vi "SCMP CoMP-S Mechanism - Diffuser.vi"(8 "error in (no error)":errorcluster, 9 "Auto Motors":bool, 10 "Old Diffuser":T1=enum."In Beam", 11 "Desired Diffuser":T1=enum."In Beam") -> (0 "error out":errorcluster, 3 "New Diffuser":T1=enum."In Beam")   [LabVIEW 2014]
uses:
  Controls/Diffuser.ctl
panel:
  # "Moving Diffuser\n    wait please"
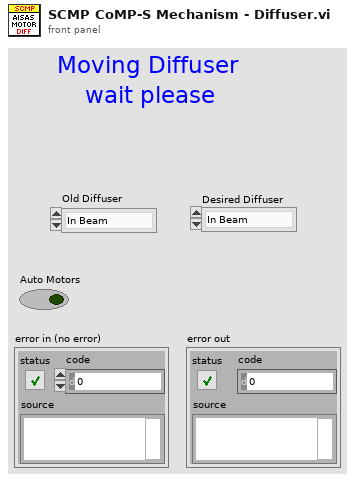
[diagram p1: front panel]
types:
  T1 = typedef "Diffuser.ctl" = enum16{"Out of Beam", "In Beam"}
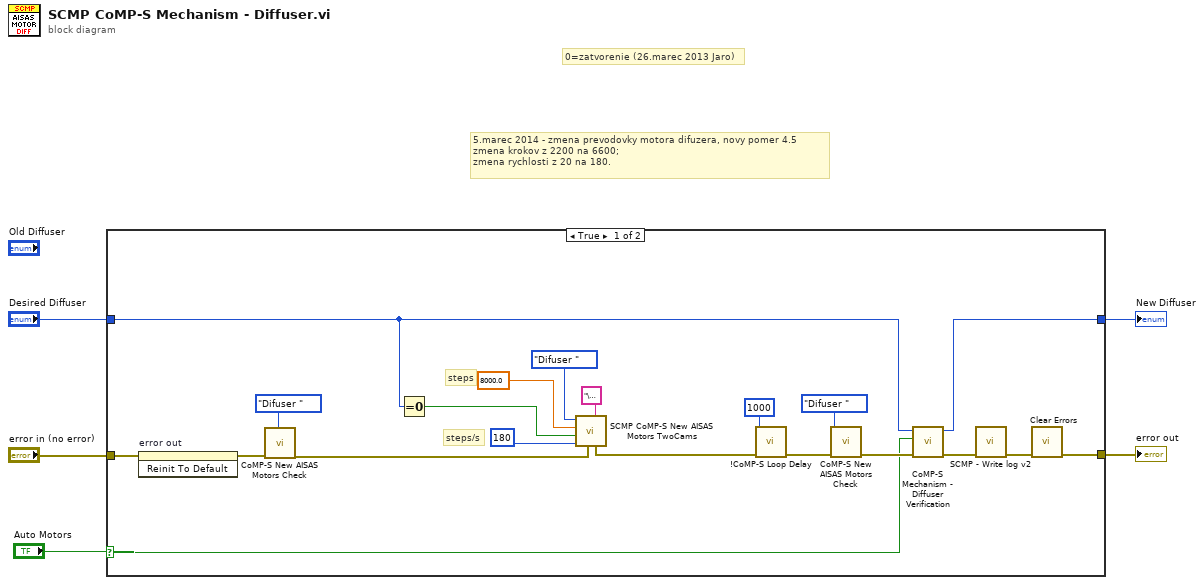
[diagram p0: block diagram]
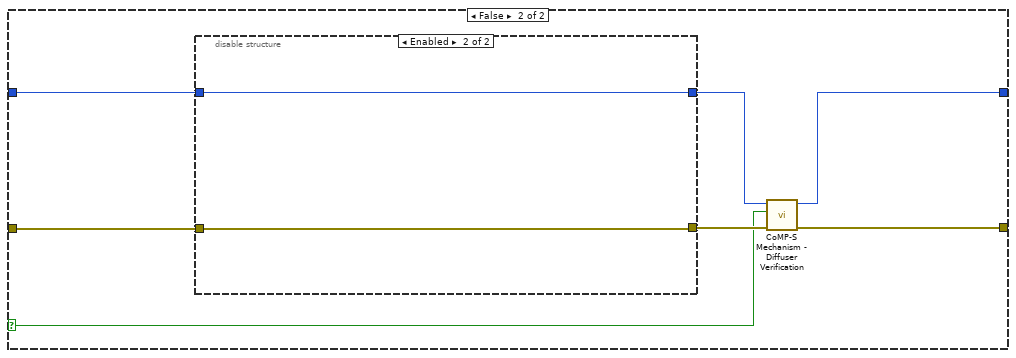
[diagram p2: hidden frame]
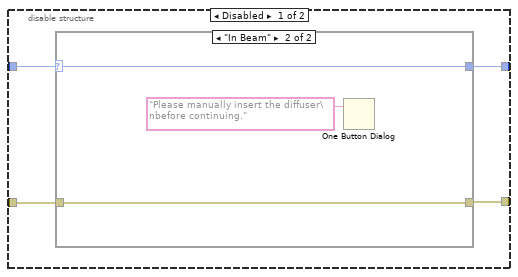
[diagram p3: hidden frame]
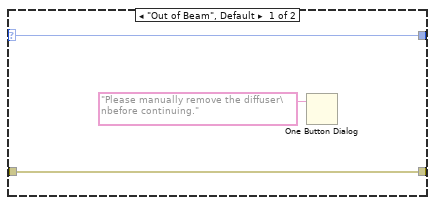
[diagram p4: hidden frame]
diagram:
  # "0=zatvorenie (26.marec 2013 Jaro)"
  # "5.marec 2014 - zmena prevodovky motora difuzera, novy pomer 4.5\nzmena krokov z 2200 na 6600;\nzmena rychlosti z 20 na 180."
  n1 = case shown="True" "Auto Motors" {
    selector: "Auto Motors" -> [w18 w26]
    tunnel: "error in (no error)" -> [w17 w32]
    tunnel: [w13 w29] -> w3
    tunnel: [w15 w27] -> w1
    tunnel: "Desired Diffuser" -> [w7 w31]
    frame True {
      # "steps/s"
      # "steps"
      n2 = invoke on="error out" class="Clust (strict)" method="Reinit To Default"(error in=w17) -> (error out=w16:errorcluster)  [unwired: 2 in, 2 out]
      n3 = call "CoMP-S New AISAS Motors Check.vi"("error in (no error)"=w16, "Motor selection"=enum32{"Rotation", "Difuser ", "Objective Lens"}."Difuser ") -> ("error out"=w20:errorcluster)  [unwired: 9 in]
      n4 = Equal To 0?(x=w7) -> (x = 0?=w6:bool)
      n5 = call "SCMP CoMP-S New AISAS Motors TwoCams.vi"("Motion Code"="\u0002", "error in (no error)"=w20, "steps/sec"=u32 180, "motor rotation"=w6, "Steps"=8000.0, "Motor selection"=enum32{"Rotation", "Difuser ", "Objective Lens"}."Difuser ") -> ("error out"=w21:errorcluster)  [unwired: 2 in, 3 out]
      n6 = call "!CoMP-S Loop Delay.vi"("error in (no error)"=w21, "Delay (2000ms)"=1000) -> ("error out"=w23:errorcluster)  [unwired: 9 in]
      n7 = call "CoMP-S New AISAS Motors Check.vi"("error in (no error)"=w23, "Motor selection"=enum32{"Rotation", "Difuser ", "Objective Lens"}."Difuser ") -> ("error out"=w19:errorcluster)  [unwired: 9 in]
      n8 = call "CoMP-S Mechanism - Diffuser Verification.vi"("error in (no error)"=w19, "Motors"=w18, "Diffuser"=w7) -> ("error out"=w14:errorcluster, "Diffuser out"=w15:T1)  [unwired: 7 in]
      n9 = call "SCMP - Write log v2.vi"("Error to log"=w14) -> ("error out"=w12:errorcluster)  [unwired: 8 in, 2 out]
      n10 = call <vilib>:"Clear Errors.vi"("error in (no error)"=w12) -> ("error out"=w13:errorcluster)  [unwired: 5 in, 1 out]
    }
    frame False {
      n11 = disable-structure shown="Enabled" {
        disable-tunnel: w32 -> [w36 w43]
        disable-tunnel: w31 -> [w35 w44]
        disable-tunnel: [w34 w43] -> w30
        disable-tunnel: [w33 w44] -> w28
        frame Disabled {
          n12 = case shown="\"In Beam\"" w35 {
            selector: w35 -> [w37 w41]
            tunnel: w36 -> [w39 w42]
            tunnel: [w39 w42] -> w34
            tunnel: [w37 w41] -> w33
            frame "Out of Beam", Default {
              n13 = One Button Dialog(message="Please manually remove the diffuser\nbefore continuing.") -> ()  [unwired: 1 in, 1 out]
            }
            frame "In Beam" {
              n14 = One Button Dialog(message="Please manually insert the diffuser\nbefore continuing.") -> ()  [unwired: 1 in, 1 out]
            }
          }
        }
        frame Enabled {
        }
      }
      n15 = call "CoMP-S Mechanism - Diffuser Verification.vi"("error in (no error)"=w30, "Motors"=w26, "Diffuser"=w28) -> ("error out"=w29:errorcluster, "Diffuser out"=w27:T1)  [unwired: 7 in]
    }
  }
  "error out" <- w3
  "New Diffuser" <- w1
